vi "SaveCluster.vi"(1 "selected path":path, 2 "Datenspeicher":refnum<vi>) -> (0 "Kein Fehler":bool)   [LabVIEW 2014]
uses:
  <vilib>/Utility/xml.llb/Write to XML File(string).vi
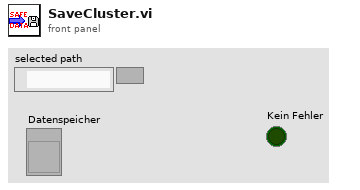
[diagram p1: front panel]
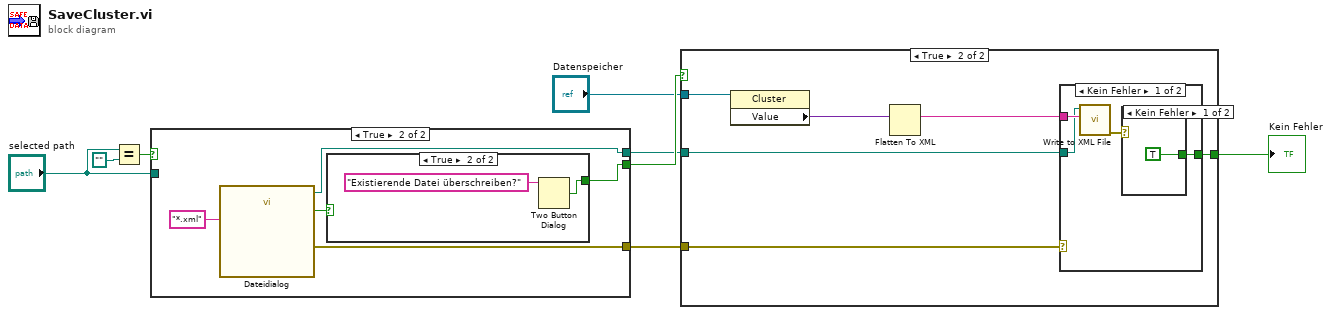
[diagram p0: block diagram]
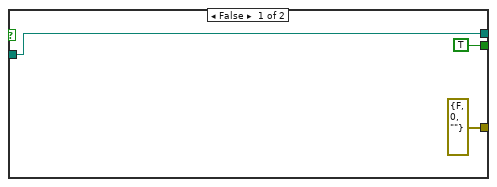
[diagram p2: hidden frame]
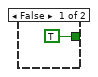
[diagram p3: hidden frame]
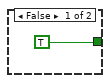
[diagram p4: hidden frame]
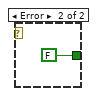
[diagram p5: hidden frame]
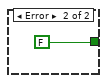
[diagram p6: hidden frame]
diagram:
  n1 = Equal?(x="selected path", y=path "") -> (x = y?=w5:bool)
  n2 = case shown="True" w5 {
    tunnel: [TRUE ("T button?") w16] -> w8
    tunnel: [errorcluster {"status"=FALSE, "code"=0, "source"=""} ("error out") w14] -> w7
    tunnel: [w10 w13] -> w6
    tunnel: "selected path" -> [w10 _]
    frame False {
    }
    frame True {
      n3 = call "Dateidialog"("pattern (all files)"="*.xml") -> ("selected path"=w13:path, "exists"=w15:bool, "error out"=w14:errorcluster)  [unwired: 11 in, 1 out]
      n4 = case shown="True" w15 {
        tunnel: [TRUE ("T button?") w18] -> w16
        frame False {
        }
        frame True {
          n5 = Two Button Dialog(message="Existierende Datei überschreiben?" ("Nachricht")) -> (T button?=w18:bool)  [unwired: 2 in]
        }
      }
    }
  }
  n6 = case shown="True" w8 {
    tunnel: w6 -> [_ w26]
    tunnel: w7 -> [_ w25]
    tunnel: "Datenspeicher" -> [_ w22]
    tunnel: [TRUE w23] -> w2
    frame False {
    }
    frame True {
      n7 = property class="Cluster"(reference=w22) -> ("Value"=w21:variant)  [unwired: 1 in, 2 out]
      n8 = Flatten To XML(anything=w21) -> (xml string=w24:string)
      n9 = case shown="Kein Fehler" w25 {
        tunnel: w24 -> [w30 _]
        tunnel: w26 -> [w28 _]
        tunnel: [w27 FALSE] -> w23
        frame No Error {
          n10 = call-poly <vilib>:"Write to XML File.vi"("XML Input"=w30, "XML File Path"=w28) -> ("error out"=w29:errorcluster)  [unwired: 7 in, 2 out]
          n11 = case shown="Kein Fehler" w29 {
            tunnel: [TRUE FALSE] -> w27
            frame No Error {
            }
            frame Error {
            }
          }
        }
        frame Error {
        }
      }
    }
  }
  "Kein Fehler" <- w2
